vi "Read Parent.vi"(8 "Error In":errorcluster, 11 "Root In":refnum<class "Root.lvclass">) -> (0 "Error Out":errorcluster, 2 "Parent":refnum<class "Abstract.lvclass">, 3 "Root Out":refnum<class "Root.lvclass">)   [LabVIEW 2018, in "Toolkit.lvlib" / "Nodes.lvlib" / "Root.lvclass"]
uses:
  Root.lvclass
  D:/Users/cfield/Code/Field R&D Services/Mustache/trunk/src/Toolkit/Low-Level/Nodes/Abstract/Abstract.lvclass
  Abstract/Abstract.lvclass
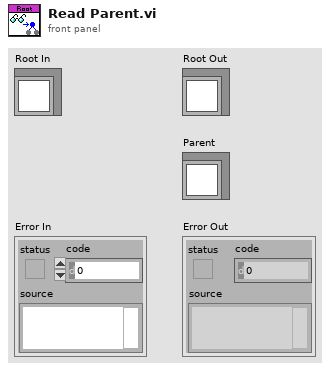
[diagram p1: front panel]
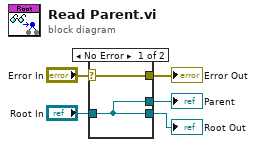
[diagram p0: block diagram]
diagram:
  n1 = case shown="No Error" "Error In" {
    selector: "Error In" -> [w7 w8]
    tunnel: [w7 w8] -> w4
    tunnel: "Root In" -> [w6 w9]
    tunnel: [w6 w9] -> w2
    tunnel: [w6 _] -> w1
    frame No Error {
    }
    frame Error {
    }
  }
  "Error Out" <- w4
  "Root Out" <- w2
  "Parent" <- w1
